vi "Read Operation Selection Rule.vi"(8 "error in (no error)":errorcluster, 11 "Scheduler in":refnum<class "Scheduler.lvclass">) -> (0 "error out":errorcluster, 2 "Operation Seletion Rule":T1=enum."SPT", 3 "Scheduler out":refnum<class "Scheduler.lvclass">)   [LabVIEW 2013, in "Scheduler.lvclass"]
uses:
  Scheduler.lvclass
  Modified GT Active Scheduler/Operation Selection Rule from Subset to Schedule.ctl
  Scheduler.lvclass/Scheduler.ctl
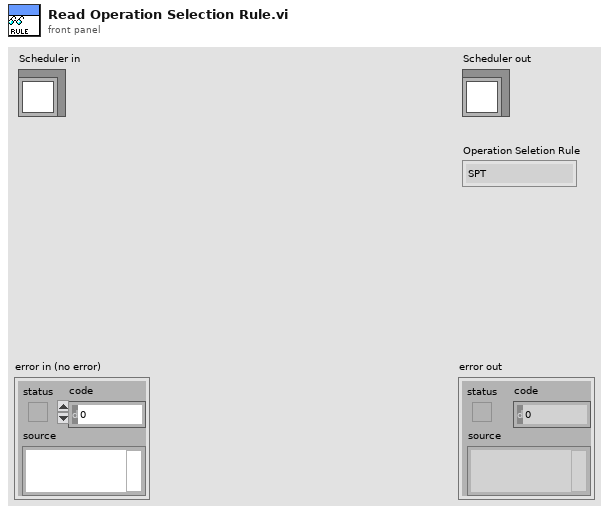
[diagram p1: front panel]
types:
  T1 = typedef "Scheduler.lvclass/Operation Selection Rule from Subset to Schedule.ctl" = enum16{"First Operation in Order", "SPT", "EDD", "MDD"}
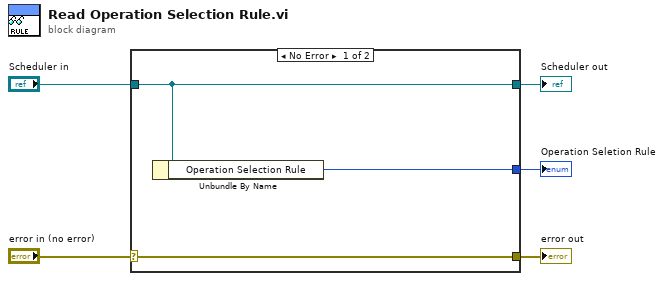
[diagram p0: block diagram]
diagram:
  n1 = case shown="No Error" "error in (no error)" {
    selector: "error in (no error)" -> [w8 w9]
    tunnel: [w8 w9] -> w4
    tunnel: [w7 w10] -> w2
    tunnel: "Scheduler in" -> [w7 w10]
    tunnel: [w6 _] -> w1
    frame No Error {
      n2 = Unbundle By Name(w7) -> ("Operation Selection Rule"=w6:T1)
    }
    frame Error {
    }
  }
  "error out" <- w4
  "Scheduler out" <- w2
  "Operation Seletion Rule" <- w1
